vi "BRig_dataLC_Loop1_T.vi"() -> (2 "output_Loop1_T":i32)   [LabVIEW 2014]
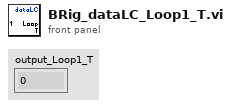
[diagram p1: front panel]
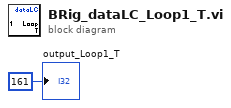
[diagram p0: block diagram]
diagram:
  "output_Loop1_T" <- 161 ("output_iBlock")
